vi "File.CSV, Read Name Value, NumInt.vi"(8 "error in":errorcluster, 9 "Default Val":i32[](array[numeric]), 10 "Names":string[](array[string]), 11 "CSV File":path) -> (0 "error out":errorcluster, 1 "Values Out":i32[](array[numeric]), 2 "Names Out":string[](array[string]))   [LabVIEW 2024]
uses:
  <vilib>/KATE/Files/File Utils.lvlib
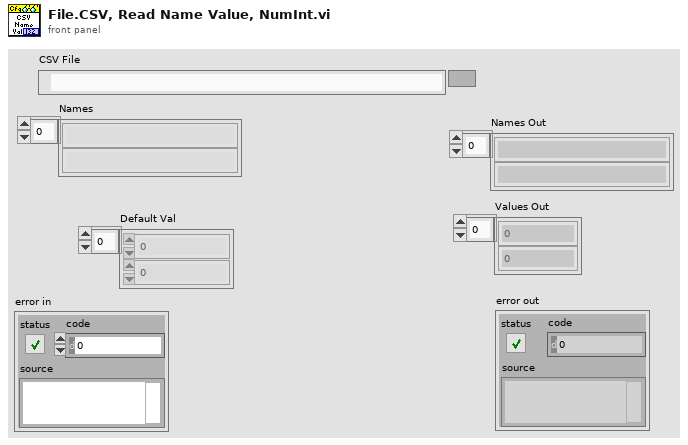
[diagram p1: front panel]
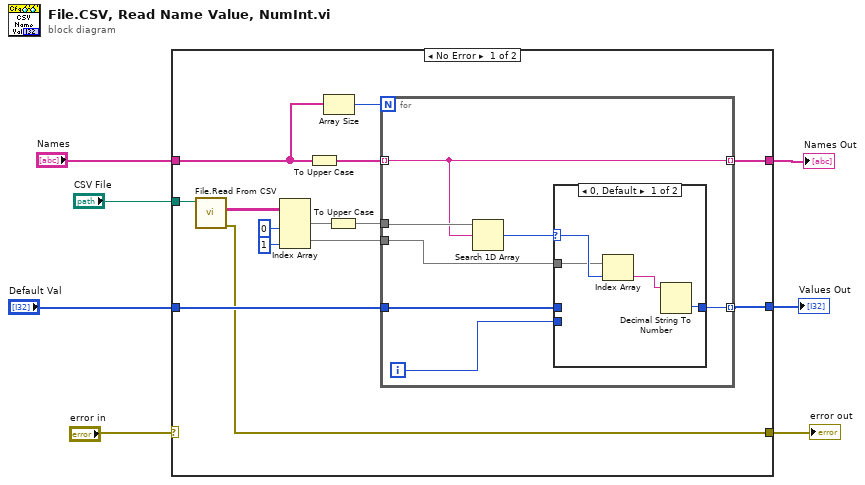
[diagram p0: block diagram]
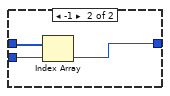
[diagram p2: hidden frame]
diagram:
  n1 = case shown="No Error" "error in" {
    selector: "error in" -> [_ w38]
    tunnel: "CSV File" -> [w21 _]
    tunnel: "Default Val" -> [w16 w36]
    tunnel: "Names" -> [w9 w37]
    tunnel: [w12 w37] -> w5
    tunnel: [w11 w36] -> w4
    tunnel: [w10 w38] -> w2
    frame No Error {
      n2 = call <vilib>:"File.Read From CSV.vi"("File"=w21) -> ("error out"=w10:errorcluster, "Data"=w20:string[][])  [unwired: 8 in, 1 out]
      n3 = Index Array(array=w20, index (col) #1=0 ("disabled index (col)"), index (col) #2=1 ("index (col)")) -> (element #1=w15:string[], element #2=w17:string[])  [unwired: 2 in]
      n4 = To Upper Case(1:w9) -> (0:w14:string[])
      n5 = Array Size(array=w9) -> (size(s)=w8:i32)
      n6 = To Upper Case(1:w15) -> (0:w13:string[])
      n7 = for {
        N: w8 -> [_]
        tunnel: w17 -> [w23]
        tunnel: w16 -> [w26]
        tunnel: w14 -> [w24] mode=indexing
        tunnel: w13 -> [w28]
        tunnel: [w25] -> w11 mode=indexing
        tunnel: [w24] -> w12 mode=indexing
        i -> [w22]
        n8 = Search 1D Array(1D array=w28, element=w24) -> (index of element=w27:i32)  [unwired: 1 in]
        n9 = case shown="0, Default" w27 {
          selector: w27 -> [w32 _]
          tunnel: w26 -> [_ w35]
          tunnel: [w30 w33] -> w25
          tunnel: w23 -> [w31 _]
          tunnel: w22 -> [_ w34]
          frame 0, Default {
            n10 = Index Array(array=w31, index=w32) -> (element=w29:string)
            n11 = Decimal String To Number(string=w29) -> (number=w30:i32)  [unwired: 2 in, 1 out]
          }
          frame -1 {
            n12 = Index Array(array=w35, index=w34) -> (element=w33:i32)
          }
        }
      }
    }
    frame Error {
    }
  }
  "Values Out" <- w4
  "Names Out" <- w5
  "error out" <- w2
